vi "getData_v6.vi"() -> ()   [LabVIEW 2014]
uses:
  <vilib>/FPGAPlugInAG/cRIO-9039/niLvFpga_Open_cRIO-9039.vi
  <vilib>/Utility/error.llb/Error Cluster From Error Code.vi
  <vilib>/rvi/errors/niLvFpgaAdjustHostInterfaceError.vi
  <vilib>/Utility/file.llb/Write To Spreadsheet File (DBL).vi
  <vilib>/FPGAPlugInAG/cRIO-9039/niLvFpga_Close_cRIO-9039.vi
  <vilib>/rvi/interface/nirviOpenFPGA/nirviOpenFPGA.xnode
  FPGA Bitfiles/test0304_FPGATarget_imptestv52_6hSeqTZk4iI.lvbitx
  FPGA VIs/imp_test_v5.vi
  <vilib>/rvi/interface/nirviMethod/nirviMethod.xnode
  <vilib>/rvi/interface/nirviCloseFPGA/nirviCloseFPGA.xnode
  <vilib>/FPGAPlugInAG/cRIO-9039/niLvFpga_ReadFifo_cRIO-9039.vi
  <vilib>/rvi/errors/niLvFpgaMergeErrorWithErrorCode.vi
panel:
  in  "File path_p":path
  in  "File path_y":path
  out "Timer (Sec)":u32
  out "FIFO empty":bool
  out "Elements Remaining":u32=10000
  in  "Time_read":i32=10000
  out "message":string=" INSTRUCTIONS:\r\rNormal Use:  When using subVIs that incorporate the error in/error out (or error I/O) structure, place this handler where you want to inform the user of an error, typically at the end of the I/O data path, as the last action of the program.  If the error in error? is ERROR, the handler creates a message describing the error and its source.  If the type of dialog = 1 (default), the message is displayed to the user, who can only acknowedge it.  If the type = 2, the user can acknowledge the message or abort execution; aborting a program with active I/O is not recommended.  If the type = 0, no message is displayed; this is used to process the error programmatically, and the error out cluster elements are wired to individual terminals for that reason.  \r\rOther Use:\n\r\nlocal testing.  To test the error code of a subVI or function that does not have the error I/O structure, you can wire its error code and a source string to the local error code and error source inputs.  If error in error? indicates no error and error code is not equal to 0, the local code and source are substituted for the error in values, and error? is set TRUE (ERROR)."
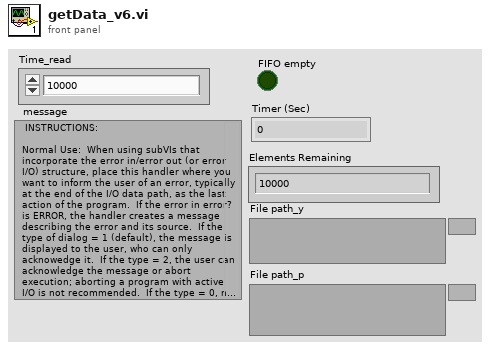
[diagram p1: front panel]
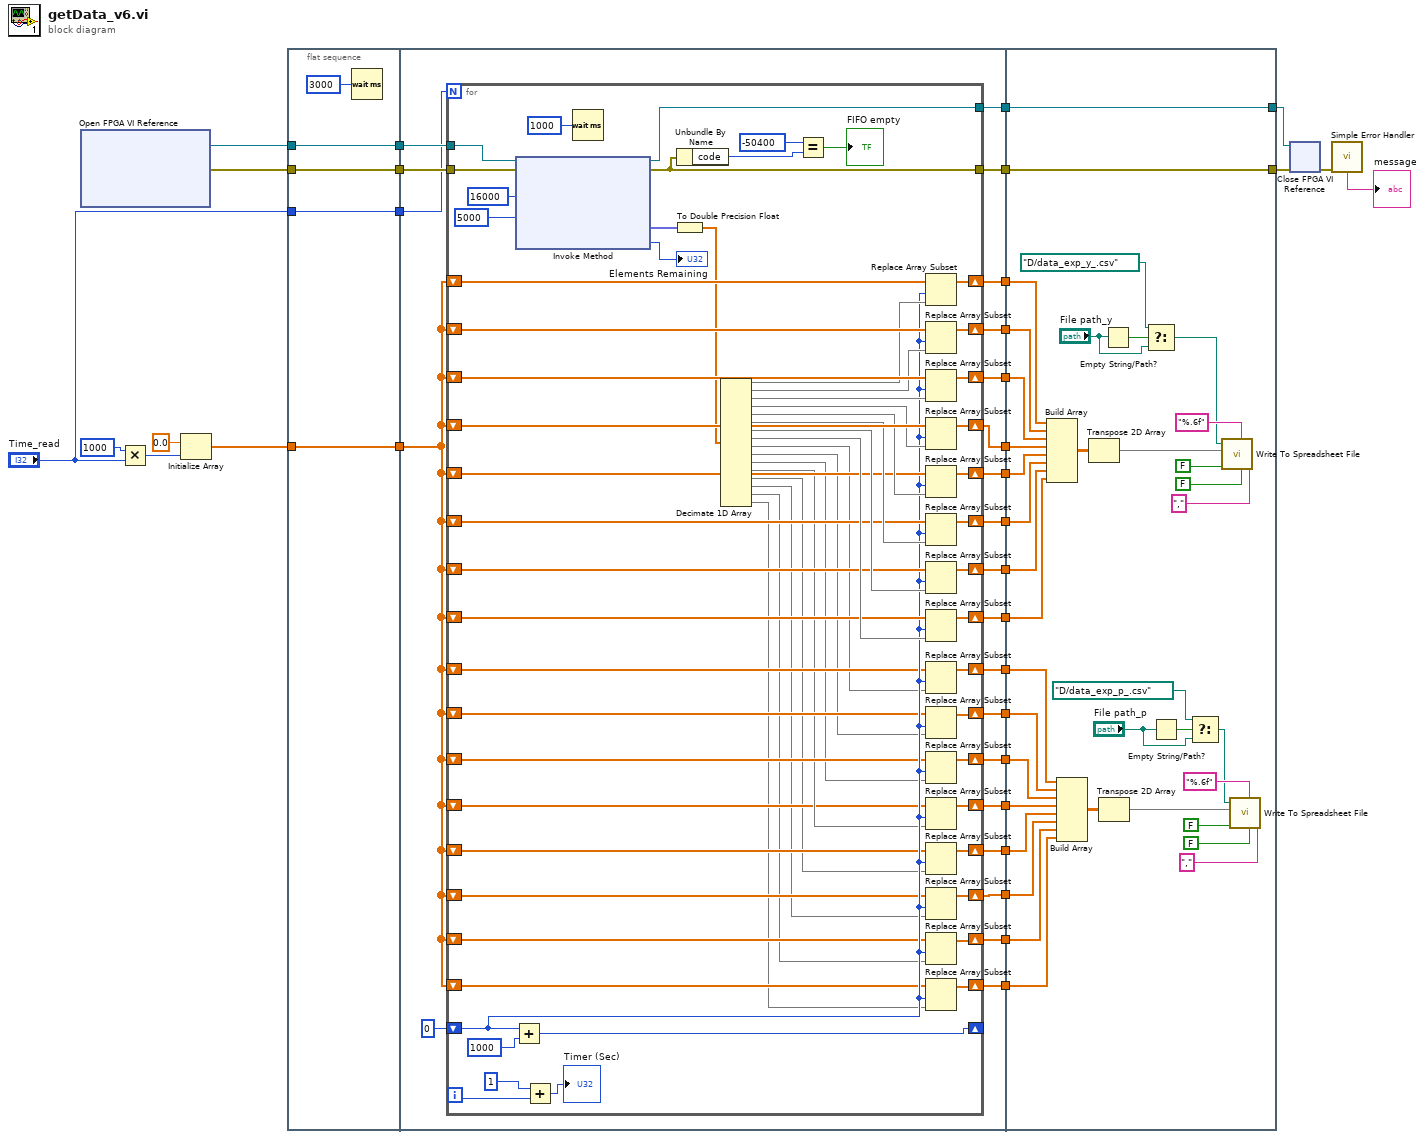
[diagram p0: block diagram]
diagram:
  n1 = xnode "Open FPGA VI Reference"() -> ("FPGA VI Reference Out"=w11:refnum<k20>, "error out"=w12:errorcluster)  [unwired: 2 in]
  n2 = Multiply(x=1000 ("y"), y="Time_read") -> (x*y=w28:i32)
  n3 = Initialize Array(0.0 ("element"), w28) -> (w30:dbl[])
  n4 = flat-sequence {
    tunnel: "Time_read" -> [w35]
    tunnel: w12 -> [w36]
    tunnel: w11 -> [w37]
    tunnel: w30 -> [w38]
    tunnel: [w38] -> w16
    tunnel: [w37] -> w15
    tunnel: [w36] -> w14
    tunnel: [w35] -> w13
    tunnel: [w58] -> w26
    tunnel: [w57] -> w25
    tunnel: [w56] -> w24
    tunnel: [w55] -> w23
    tunnel: [w54] -> w22
    tunnel: [w53] -> w21
    tunnel: [w52] -> w20
    tunnel: [w51] -> w19
    tunnel: [w50] -> w18
    tunnel: [w49] -> w17
    tunnel: w16 -> [w39]
    tunnel: w15 -> [w60]
    tunnel: w14 -> [w59]
    tunnel: w13 -> [w48]
    tunnel: [w47] -> w10
    tunnel: [w46] -> w9
    tunnel: [w45] -> w8
    tunnel: [w44] -> w7
    tunnel: [w43] -> w6
    tunnel: [w42] -> w5
    tunnel: [w41] -> w4
    tunnel: [w40] -> w3
    tunnel: w26 -> [w163]
    tunnel: w25 -> [w162]
    tunnel: w24 -> [w161]
    tunnel: [w166] -> w2
    tunnel: w23 -> [w166]
    tunnel: [w165] -> w1
    tunnel: w22 -> [w165]
    tunnel: w21 -> [w160]
    tunnel: w20 -> [w159]
    tunnel: w19 -> [w157]
    tunnel: w18 -> [w158]
    tunnel: w17 -> [w164]
    tunnel: w10 -> [w150]
    tunnel: w9 -> [w149]
    tunnel: w8 -> [w148]
    tunnel: w7 -> [w147]
    tunnel: w6 -> [w146]
    tunnel: w5 -> [w145]
    tunnel: w4 -> [w144]
    tunnel: w3 -> [w143]
    frame #0 {
      n5 = Wait (ms)(milliseconds to wait=u32 3000 ("y")) -> ()  [unwired: 1 out]
    }
    frame #1 {
      n6 = for {
        N: w48 -> [_]
        shift-right: [w126] -> _
        shift-left: 0 -> [w88]
        shift-right: [w115] -> w58
        shift-left: w39 -> [w124]
        shift-right: [w114] -> w57
        shift-left: w39 -> [w123]
        shift-right: [w113] -> w56
        shift-left: w39 -> [w122]
        shift-right: [w116] -> w49
        shift-left: w39 -> [w125]
        tunnel: w60 -> [w87]
        tunnel: w59 -> [w86]
        tunnel: [w94] -> w55
        tunnel: [w95] -> w54
        shift-right: [w107] -> w53
        shift-left: w39 -> [w108]
        shift-right: [w105] -> w52
        shift-left: w39 -> [w106]
        shift-right: [w104] -> w50
        shift-left: w39 -> [w103]
        shift-right: [w101] -> w51
        shift-left: w39 -> [w102]
        shift-right: [w78] -> w47
        shift-left: w39 -> [w77]
        shift-right: [w79] -> w46
        shift-left: w39 -> [w76]
        shift-right: [w80] -> w45
        shift-left: w39 -> [w75]
        shift-right: [w81] -> w44
        shift-left: w39 -> [w66]
        shift-right: [w82] -> w43
        shift-left: w39 -> [w74]
        shift-right: [w83] -> w42
        shift-left: w39 -> [w73]
        shift-right: [w84] -> w41
        shift-left: w39 -> [w72]
        shift-right: [w85] -> w40
        shift-left: w39 -> [w71]
        i -> [w91]
        n7 = Add(x=w88, y=1000) -> (x+y=w126:i32)
        n8 = xnode "Invoke Method"("FPGA VI Reference In"=w87, "error in"=w86, "Number of Elements"=u32 16000, "Timeout (ms)"=5000) -> ("FPGA VI Reference Out"=w94:refnum<k20>, "error out"=w95:errorcluster, "Data"=w92:fxp<+/-,45,25>[], "Elements Remaining"=→"Elements Remaining":u32)
        n9 = Add(x=1, y=w91) -> (x+y=→"Timer (Sec)":i32)
        n10 = Wait (ms)(milliseconds to wait=u32 1000 ("y")) -> ()  [unwired: 1 out]
        n11 = To Double Precision Float(number=w92) -> (double precision float=w121:dbl[])
        n12 = Unbundle By Name(w95) -> ("code"=w99:i32)
        n13 = Decimate 1D Array(w121) -> (w120:dbl[], w119:dbl[], w118:dbl[], w117:dbl[], w112:dbl[], w111:dbl[], w110:dbl[], w109:dbl[], w70:dbl[], w69:dbl[], w68:dbl[], w67:dbl[], w65:dbl[], w64:dbl[], w63:dbl[], w62:dbl[])
        n14 = Equal?(x=-50400 ("y"), y=w99) -> (x = y?=→"FIFO empty":bool)
        n15 = Replace Array Subset(array=w125, new element=w120, index=w88) -> (w116:dbl[])
        n16 = Replace Array Subset(array=w124, new element=w119, index=w88) -> (w115:dbl[])
        n17 = Replace Array Subset(array=w123, new element=w118, index=w88) -> (w114:dbl[])
        n18 = Replace Array Subset(array=w122, new element=w117, index=w88) -> (w113:dbl[])
        n19 = Replace Array Subset(array=w108, new element=w112, index=w88) -> (w107:dbl[])
        n20 = Replace Array Subset(array=w106, new element=w111, index=w88) -> (w105:dbl[])
        n21 = Replace Array Subset(array=w103, new element=w110, index=w88) -> (w104:dbl[])
        n22 = Replace Array Subset(array=w102, new element=w109, index=w88) -> (w101:dbl[])
        n23 = Replace Array Subset(array=w77, new element=w70, index=w88) -> (w78:dbl[])
        n24 = Replace Array Subset(array=w76, new element=w69, index=w88) -> (w79:dbl[])
        n25 = Replace Array Subset(array=w75, new element=w68, index=w88) -> (w80:dbl[])
        n26 = Replace Array Subset(array=w66, new element=w67, index=w88) -> (w81:dbl[])
        n27 = Replace Array Subset(array=w74, new element=w65, index=w88) -> (w82:dbl[])
        n28 = Replace Array Subset(array=w73, new element=w64, index=w88) -> (w83:dbl[])
        n29 = Replace Array Subset(array=w72, new element=w63, index=w88) -> (w84:dbl[])
        n30 = Replace Array Subset(array=w71, new element=w62, index=w88) -> (w85:dbl[])
      }
    }
    frame #2 {
      n31 = Build Array(w164, w163, w162, w161, w160, w159, w158, w157) -> (w151:dbl[][])
      n32 = Build Array(w150, w149, w148, w147, w146, w145, w144, w143) -> (w142:dbl[][])
      n33 = Transpose 2D Array(2D array=w151) -> (transposed array=w155:dbl[][])
      n34 = Transpose 2D Array(2D array=w142) -> (transposed array=w137:dbl[][])
      n35 = Empty String/Path?(string/path="File path_y") -> (empty?=w136:bool)
      n36 = Select(t=path "D:/data_exp_y_.csv" ("file path (dialog if empty)"), s=w136, f="File path_y") -> (s? t:f=w133:path)
      n37 = Empty String/Path?(string/path="File path_p") -> (empty?=w132:bool)
      n38 = Select(t=path "D:/data_exp_p_.csv" ("file path (dialog if empty)"), s=w132, f="File path_p") -> (s? t:f=w129:path)
      n39 = call-poly <vilib>:"Write To Spreadsheet File.vi"("delimiter (\\t)"="," ("delimiter (\\t)"), "transpose? (no:F)"=FALSE, "format (%.3f)"="%.6f" ("format (%d)"), "append to file? (new file:F)"=FALSE, "2D data"=w155, "file path (dialog if empty)"=w133) -> ()  [unwired: 2 in, 1 out]
      n40 = call-poly <vilib>:"Write To Spreadsheet File.vi"("delimiter (\\t)"="," ("delimiter (\\t)"), "transpose? (no:F)"=FALSE, "format (%.3f)"="%.6f" ("format (%d)"), "append to file? (new file:F)"=FALSE, "2D data"=w137, "file path (dialog if empty)"=w129) -> ()  [unwired: 2 in, 1 out]
    }
  }
  n41 = xnode "Close FPGA VI Reference"("FPGA VI Reference In"=w2, "error in"=w1) -> ("error out"=w32:errorcluster)
  n42 = call <vilib>:"Simple Error Handler.vi"("error in (no error)"=w32) -> ("message"=→"message":string)  [unwired: 4 in, 4 out]
